vi "Run.vi"(8 "error in (no error)":errorcluster, 11 "JSON Lexer in":refnum<class "JSON Lexer.lvclass">) -> (0 "error out":errorcluster, 3 "JSON Lexer out":refnum<class "JSON Lexer.lvclass">)   [LabVIEW 2020, in "JKI JSON Serialization.lvlib" / "JSON Lexer.lvclass"]
uses:
  JSON Lexer.lvclass
  JSON Lexer States.ctl
  JSON Lexer.lvclass/JSON Lexer.ctl
  <vilib>/addons/_JKI.lib/Unicode/UTF-8 String/UTF-8 String.lvclass/UTF-8 String.ctl
  Backup.vi
  Next.vi
  <vilib>/addons/_JKI.lib/Unicode/UTF-8 String/Index Rune as UTF-8 Substring.vi
  Ignore.vi
  <vilib>/addons/_JKI.lib/Unicode/UTF-8 String/Next Rune As UTF-8 Substring.vi
  <vilib>/addons/_JKI.lib/Unicode/UTF-8 String/Bytes In Rune.vi
  Emit.vi
  Accept.vi
  Accept Multiple.vi
  Match.vi
  Peek.vi
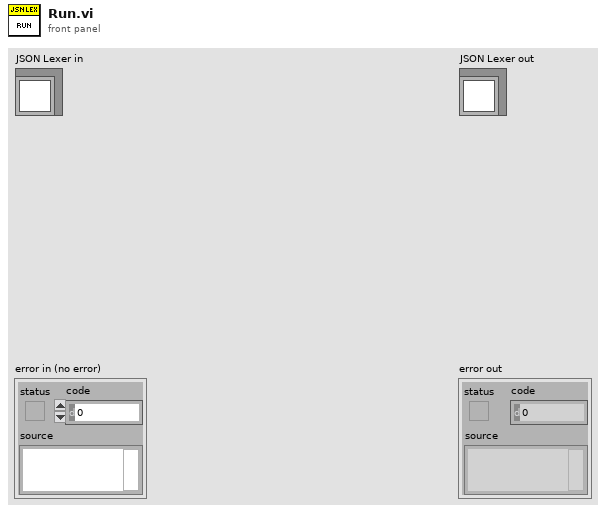
[diagram p1: front panel]
types:
  T1 = typedef "JKI JSON Serialization.lvlib/JSON Lexer.lvclass/JSON Lexer States.ctl" = enum16{"Undefined", "Value", "String", "Numeric", "Number", "Symbol", "Symbolic Number"}
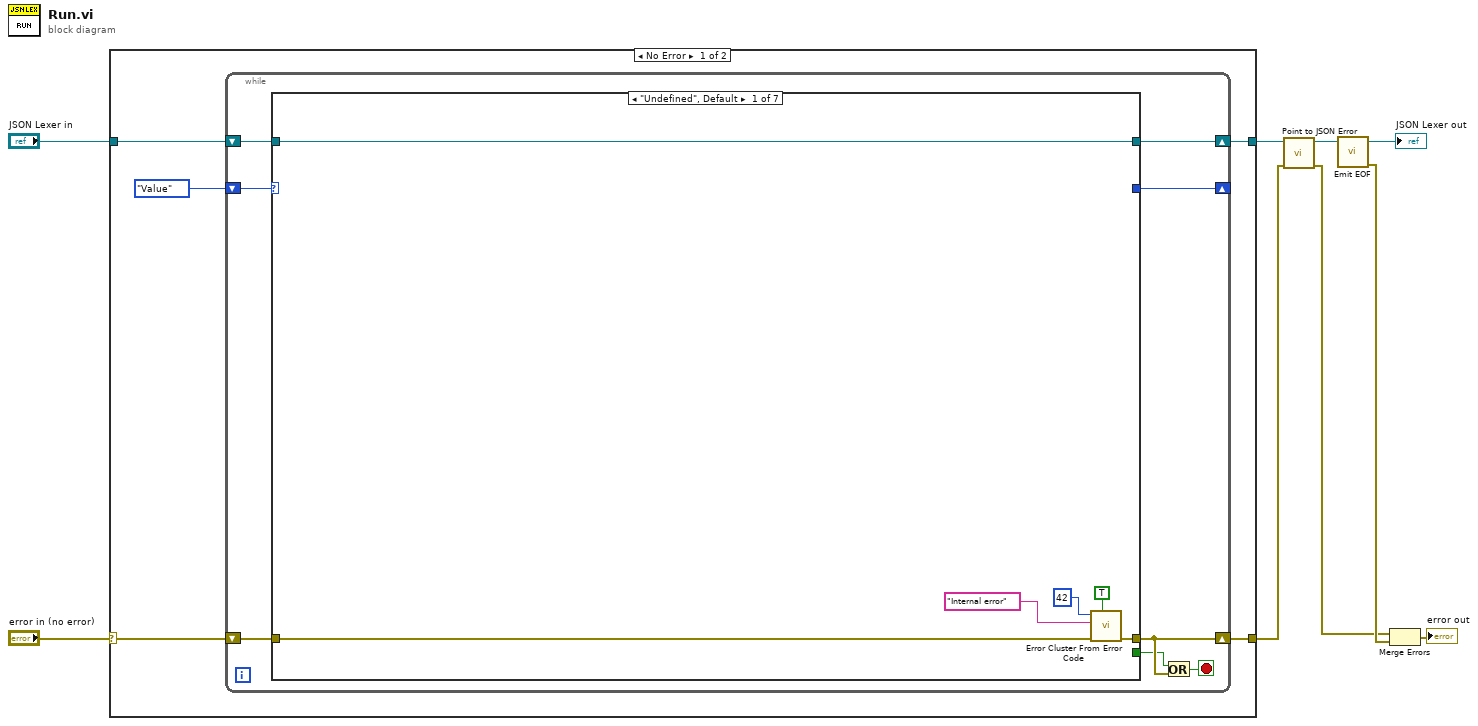
[diagram p0: block diagram]
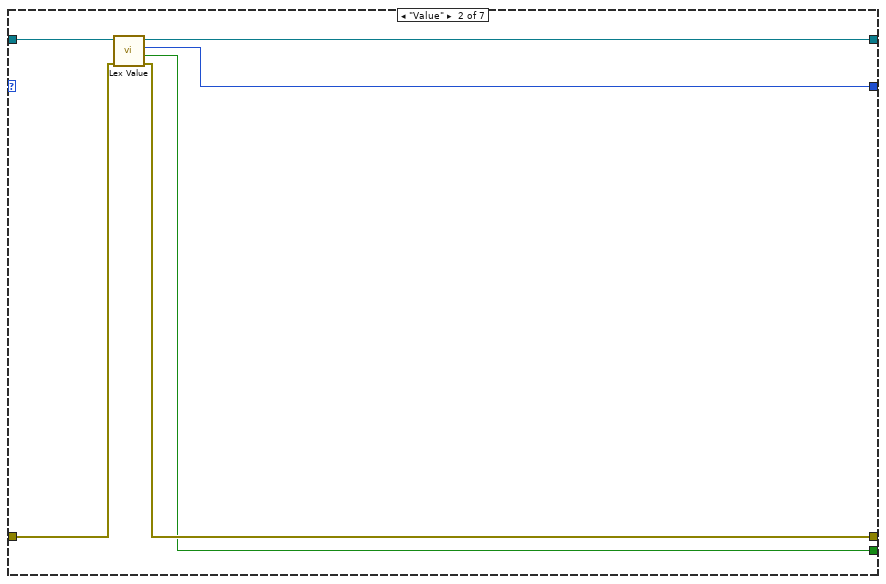
[diagram p2: hidden frame]
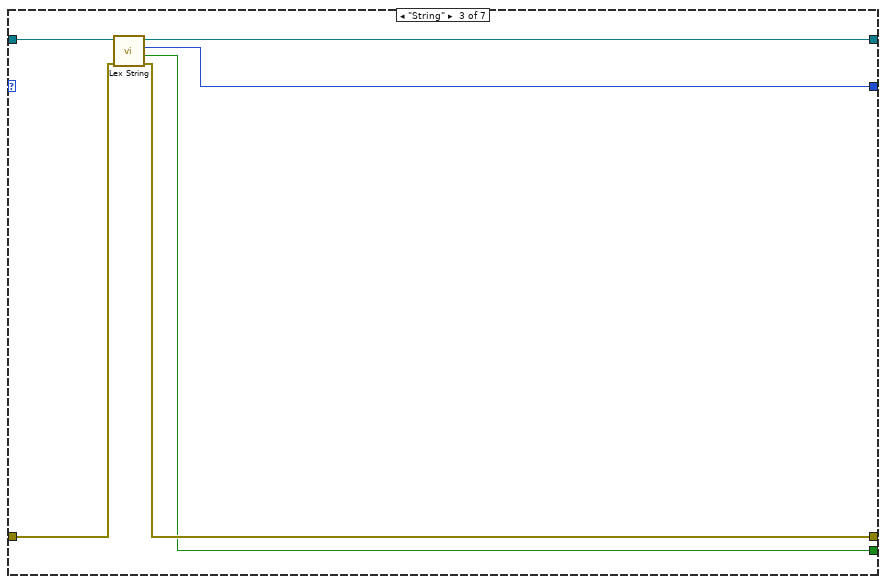
[diagram p3: hidden frame]
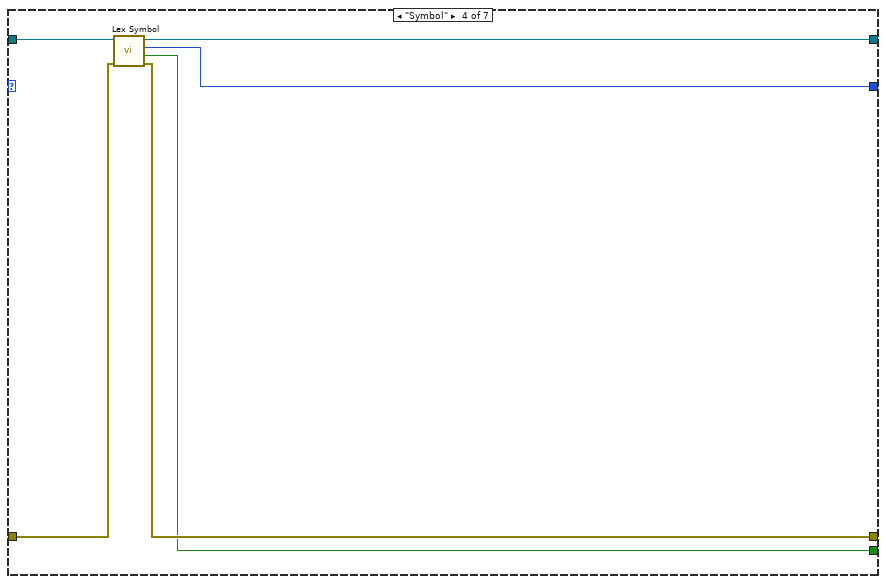
[diagram p4: hidden frame]
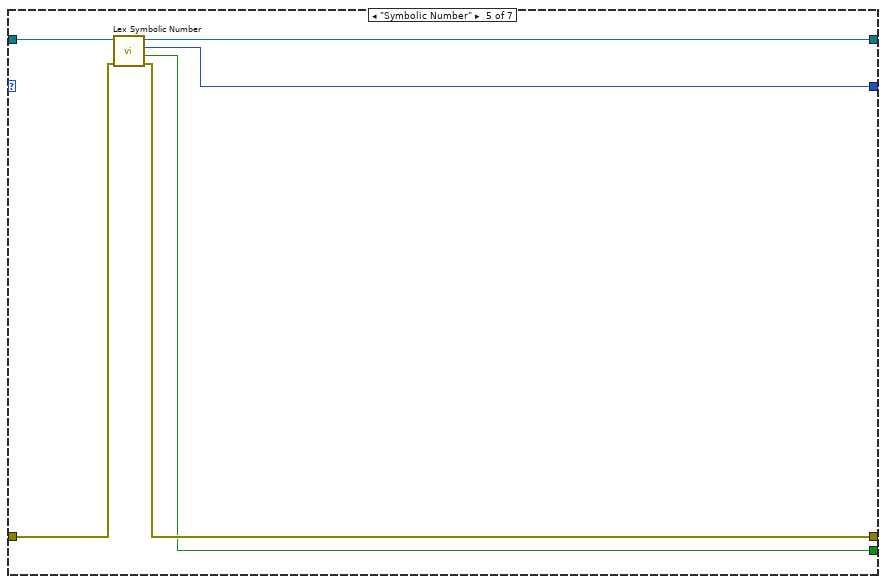
[diagram p5: hidden frame]
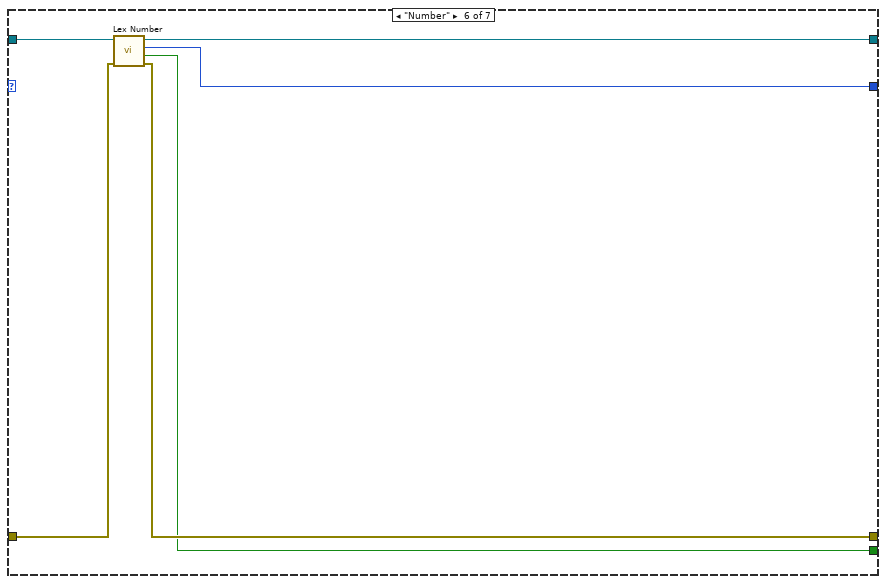
[diagram p6: hidden frame]
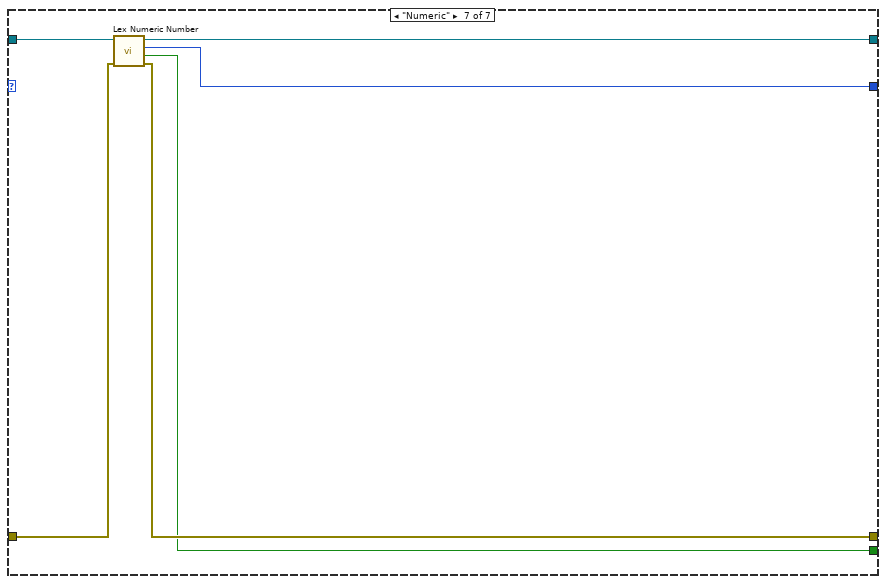
[diagram p7: hidden frame]
diagram:
  n1 = case shown="No Error" "error in (no error)" {
    selector: "error in (no error)" -> [w13 w66]
    tunnel: [w10 w66] -> w3
    tunnel: [w11 w65] -> w4
    tunnel: "JSON Lexer in" -> [w14 w65]
    frame No Error {
      n2 = while {
        shift-right: [w21] -> w11
        shift-left: w14 -> [w22]
        shift-right: [w18] -> w10
        shift-left: w13 -> [w20]
        shift-right: [w17] -> _
        shift-left: JSON_Lexer_States."Value" ("JSON Lexer State") -> [w16]
        stop <- w19 stop-if-true
        n3 = case shown="\"Undefined\", Default" w16 {
          tunnel: w22 -> [w24 w34 w40 w46 w52 w58 w64]
          tunnel: [w24 w33 w39 w45 w51 w57 w63] -> w21
          tunnel: w20 -> [w23 w32 w38 w44 w50 w56 w62]
          tunnel: [w28 w31 w37 w43 w49 w55 w61] -> w18
          tunnel: [_ w30 w36 w42 w48 w54 w60] -> w17
          tunnel: [_ w29 w35 w41 w47 w53 w59] -> w15
          frame "Undefined", Default {
            n4 = call <vilib>:"Error Cluster From Error Code.vi"("show call chain? (False)"=TRUE, "error in (no error)"=w23, "error message (\"\")"="Internal error", "error code (0)"=42) -> ("error out"=w28:errorcluster)  [unwired: 5 in]
          }
          frame "Value" {
            n5 = call "Lex Value.vi"("error in (no error)"=w32, "JSON Lexer in"=w34) -> ("error out"=w31:errorcluster, "EOF"=w29:bool, "Next State"=w30:T1, "JSON Lexer out"=w33:refnum<class "JSON Lexer.lvclass">)  [unwired: 6 in]
          }
          frame "String" {
            n6 = call "Lex String.vi"("error in (no error)"=w38, "JSON Lexer in"=w40) -> ("error out"=w37:errorcluster, "EOF"=w35:bool, "Next State"=w36:T1, "JSON Lexer out"=w39:refnum<class "JSON Lexer.lvclass">)  [unwired: 6 in]
          }
          frame "Symbol" {
            n7 = call "Lex Symbol.vi"("error in (no error)"=w44, "JSON Lexer in"=w46) -> ("error out"=w43:errorcluster, "EOF"=w41:bool, "Next State"=w42:T1, "JSON Lexer out"=w45:refnum<class "JSON Lexer.lvclass">)  [unwired: 6 in]
          }
          frame "Symbolic Number" {
            n8 = call "Lex Symbolic Number.vi"("error in (no error)"=w50, "JSON Lexer in"=w52) -> ("error out"=w49:errorcluster, "EOF"=w47:bool, "Next State"=w48:T1, "JSON Lexer out"=w51:refnum<class "JSON Lexer.lvclass">)  [unwired: 6 in]
          }
          frame "Number" {
            n9 = call "Lex Number.vi"("error in (no error)"=w56, "JSON Lexer in"=w58) -> ("error out"=w55:errorcluster, "EOF"=w53:bool, "Next State"=w54:T1, "JSON Lexer out"=w57:refnum<class "JSON Lexer.lvclass">)  [unwired: 6 in]
          }
          frame "Numeric" {
            n10 = call "Lex Numeric Number.vi"("error in (no error)"=w62, "JSON Lexer in"=w64) -> ("error out"=w61:errorcluster, "EOF"=w59:bool, "Next State"=w60:T1, "JSON Lexer out"=w63:refnum<class "JSON Lexer.lvclass">)  [unwired: 6 in]
          }
        }
        n11 = Or(x=w15, y=w18) -> (x .or. y?=w19:bool)
      }
    }
    frame Error {
    }
  }
  n12 = call "Point to JSON Error.vi"("error in (no error)"=w3, "JSON Lexer in"=w4) -> ("error out"=w2:errorcluster, "JSON Lexer out"=w1:refnum<class "JSON Lexer.lvclass">)  [unwired: 8 in]
  n13 = call "Emit EOF.vi"("JSON Lexer in"=w1) -> ("error out"=w5:errorcluster, "JSON Lexer out"=→"JSON Lexer out":refnum<class "JSON Lexer.lvclass">)  [unwired: 9 in]
  n14 = Merge Errors(w2, w5) -> (→"error out":errorcluster)
